vi "multiple_animal_parameters.vi"(9 "Input \nparameters":T3={"Frame rate (ms)"=2000, "Worm strain"="N2", "# Images"=0, "State"=enum."Image acquisition", "Time elapsed"=0.0, "Max_num_runs"=100000, "#TTL"=0, "Time of start TTL"=100000, "ImSub Value"=0, "Time of last TTL"=0, "# Animals per column"=2, "# Animals per row"=2, "# AdjacentTTL"=0, "Sleep deprivation status"="", "Sleep Detection"=FALSE, "# Sleep detections"=0, "Time of first sleep detection"=0, "Time max # adjacent TTL"=0, "Image t-1"=[], "Image t"=[]} {"# Animals per row" items=["1"=1, "2"=2, "3"=3, "4"=4]; "# Animals per column" items=["1"=1, "2"=2, "3"=3, "4"=4]}, 10 "Deprivation\nSettings":T1={"SD animal row"=0, "Kstd"=40.0, "# Images for\nsleep detection"=10, "Kmean"=1.5, "Start time of sleep detection (images):"=1000, "SD animal column"=0, "Length (images)"=3600, "# TTL"=10000, "by x images after first detection"=0, "Between TTL pulses"=0, "\nby x detections"=9, "# Total immobility\n detections"=0.0, "max # adjacent\nTTL"=0.0, "TTL x start\ntime deprivation\n"=0.0, "Max #\nadjacent TTL"=10000, " Ca2+\nmode"=0} {"SD animal column" items=["1", "2", "3", "4"]; "SD animal row" items=["1", "2", "3", "4"]}, 11 "Action":T4) -> (2 "Animal\nparameters":cluster{"# Animals":i32, "Index SD animal":i32} caption="XY-pixel\nranges")   [LabVIEW 2011]
uses:
  Action Items.ctl
  state.ctl
panel:
  in  "Animal\nparameters":cluster{"# Animals":i32, "Index SD animal":i32} caption="XY-pixel \nranges"
  # "Sleep deprivation settings"
  # "Select deprivation animal"
  # "Column"
  # "Row"
  # "Sleep detection parameters"
  # "Sleep deprivation parameters"
  # "Delay deprivation start:"
  # "Pause deprivation (images):"
  # "Stop deprivation after:"
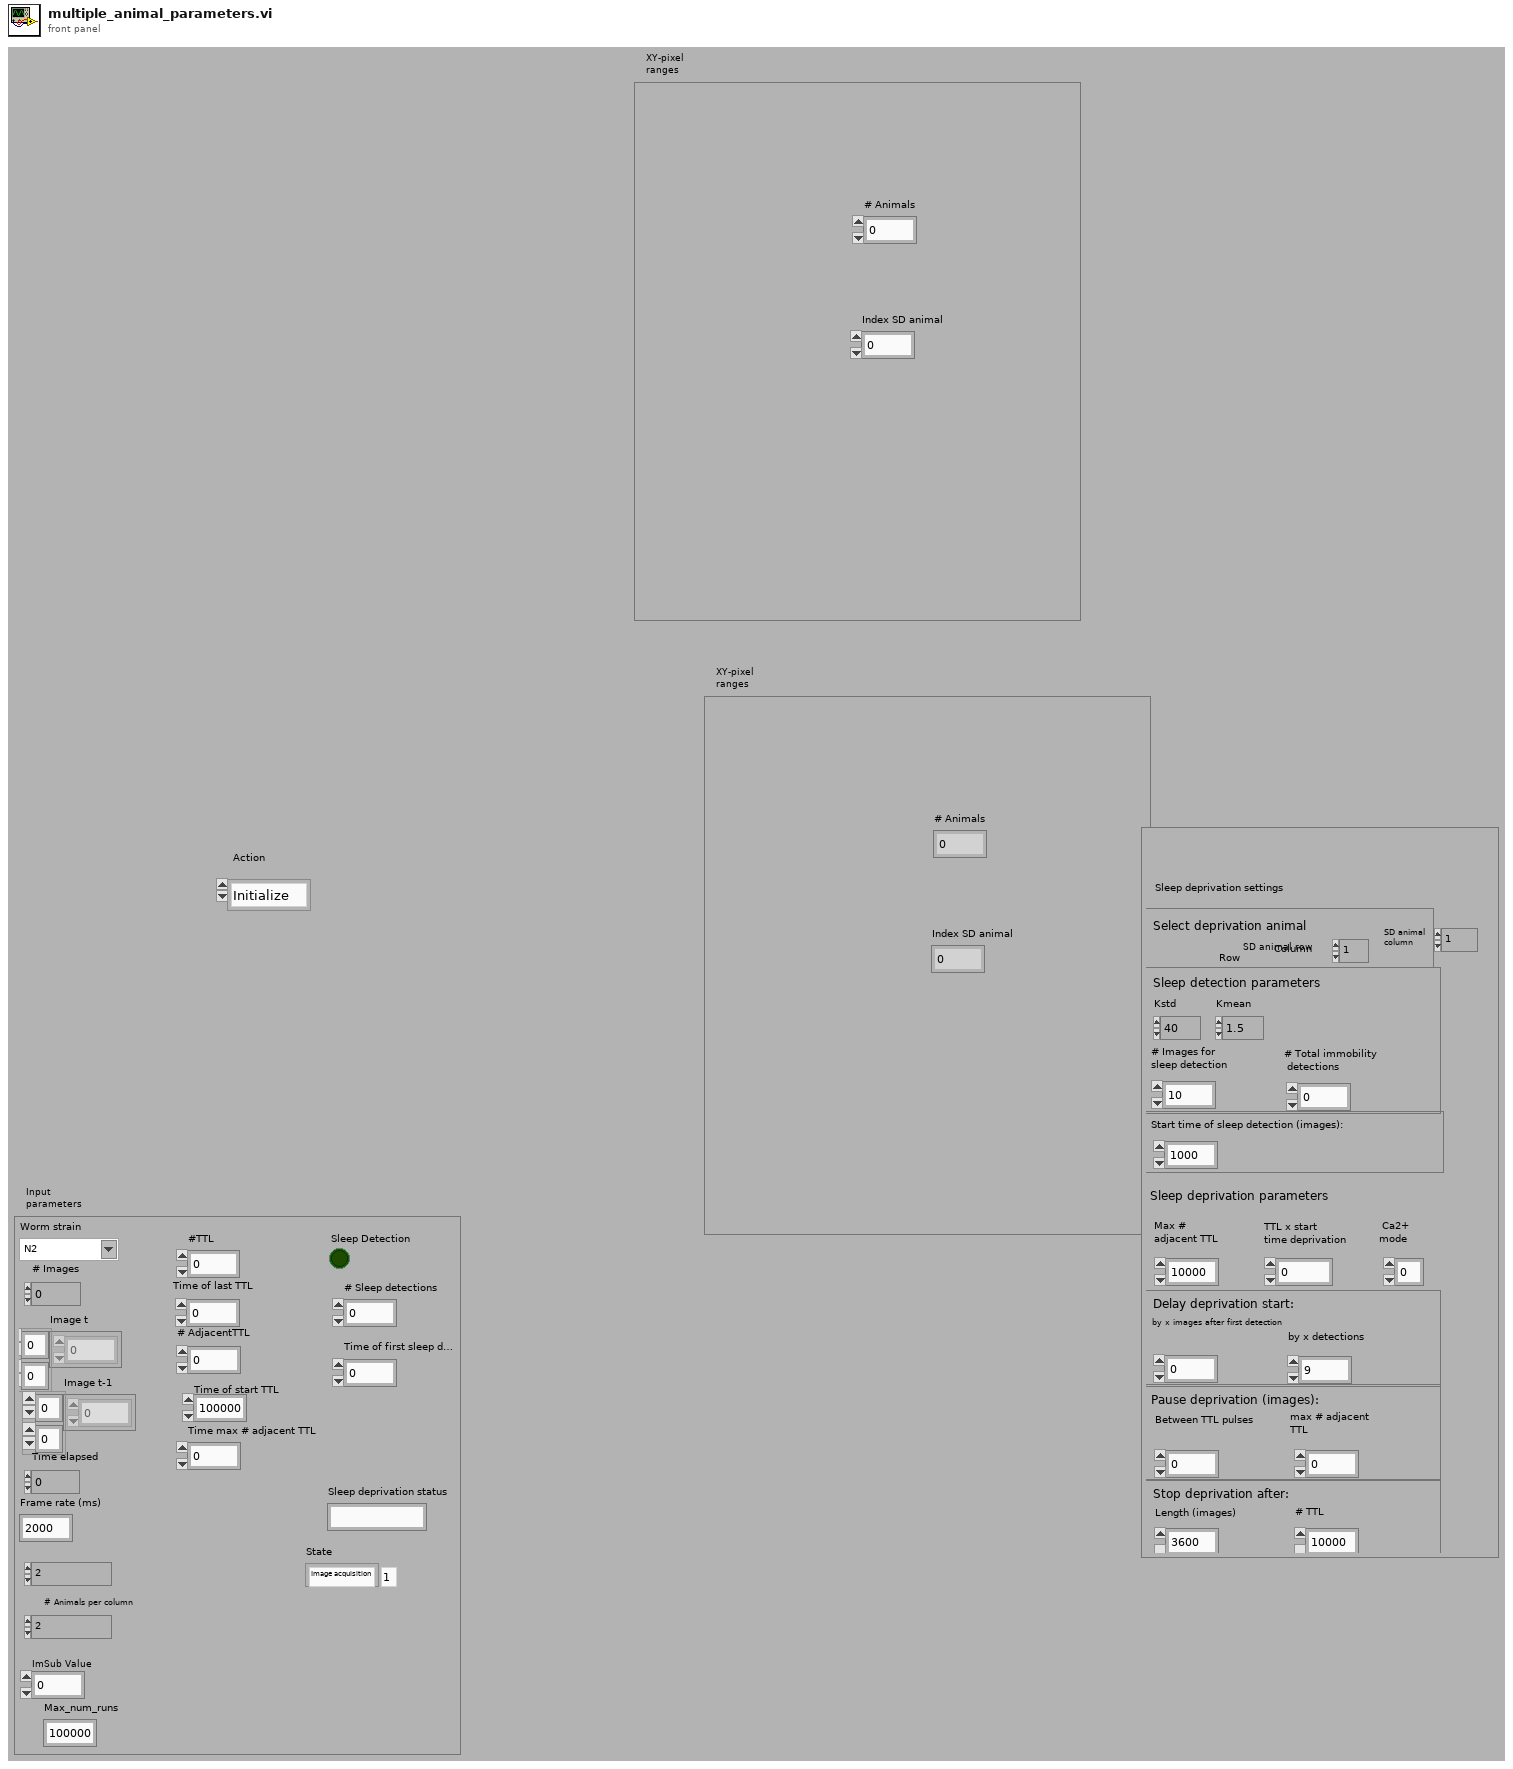
[diagram p1: front panel]
types:
  T1 = cluster{"SD animal row":u32, "Kstd":dbl, "# Images for\nsleep detection":i32, "Kmean":dbl, "Start time of sleep detection (images):":i32, "SD animal column":u32, "Length (images)":i32, "# TTL":i32, "by x images after first detection":i32, "Between TTL pulses":i32, "\nby x detections":i32, "# Total immobility\n detections":dbl, "max # adjacent\nTTL":dbl, "TTL x start\ntime deprivation\n":dbl, "Max #\nadjacent TTL":i32, " Ca2+\nmode":i32}
  T2 = typedef "state.ctl" = enum16{"Initialize measurement", "Image acquisition", "Image processing", "Sleep detection", "Control TTL protocol ", "Sleep deprivation", "Update image & exit condition", "Wait "}
  T3 = cluster{"Frame rate (ms)":u32, "Worm strain":string, "# Images":i32, "State":T2, "Time elapsed":dbl, "Max_num_runs":i32, "#TTL":i32, "Time of start TTL":i32, "ImSub Value":i32, "Time of last TTL":i32, "# Animals per column":u32, "# Animals per row":u32, "# AdjacentTTL":i32, "Sleep deprivation status":string, "Sleep Detection":bool, "# Sleep detections":i32, "Time of first sleep detection":i32, "Time max # adjacent TTL":i32, "Image t-1":i32[][], "Image t":i32[][]}
  T4 = typedef "Action Items.ctl" = enum16{"Initialize", "Get"}
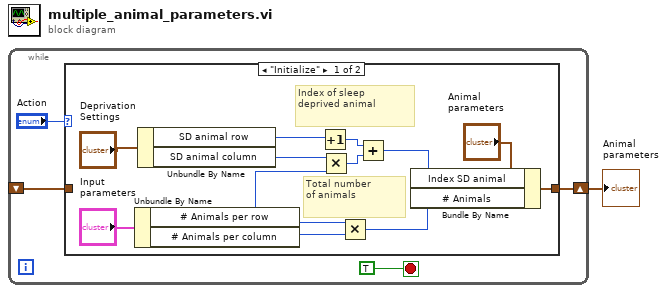
[diagram p0: block diagram]
diagram:
  n1 = while {
    shift-right: [w2] -> w1
    shift-left: _ -> [w3]
    stop <- TRUE ("stop") stop-if-true
    n2 = case shown="\"Initialize\"" "Action" {
      tunnel: w3 -> [_ w18]
      tunnel: [w9 w18] -> w2
      frame "Initialize" {
        # "Total number\nof animals"
        # "Index of sleep\ndeprived animal"
        n3 = Unbundle By Name("Input \nparameters") -> ("# Animals per row"=w14:u32, "# Animals per column"=w16:u32)
        n4 = Unbundle By Name("Deprivation\nSettings") -> ("SD animal row"=w8:u32, "SD animal column"=w7:u32)
        n5 = Increment(x=w8) -> (x+1=w6:u32)
        n6 = Multiply(x=w7, y=w14) -> (x*y=w13:u32)
        n7 = Multiply(x=w14, y=w16) -> (x*y=w11:u32)
        n8 = Add(x=w6, y=w13) -> (x+y=w12:u32)
        n9 = Bundle By Name(cluster="Animal\nparameters", "Index SD animal"=w12, "# Animals"=w11) -> (w9:cluster{"# Animals":i32, "Index SD animal":i32})
      }
      frame "Get" {
      }
    }
  }
  "Animal\nparameters" <- w1
